vi "Init.vi"(8 "error in (no error)":errorcluster, 10 "Responder names":string[](array[string]), 11 "Response Synchronizer in":refnum<class "Response Synchronizer.lvclass">) -> (0 "error out":errorcluster, 3 "Response Synchronizer out":refnum<class "Response Synchronizer.lvclass">)   [LabVIEW 2021, in "Response Synchronizer.lvclass"]
uses:
  Response Synchronizer.lvclass
  Acquired Result/Acquired Result.lvclass
  Response Synchronizer.lvclass/Response Synchronizer.ctl
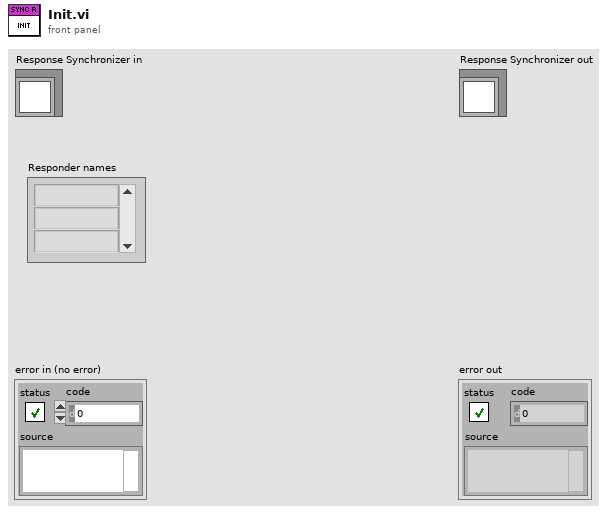
[diagram p1: front panel]
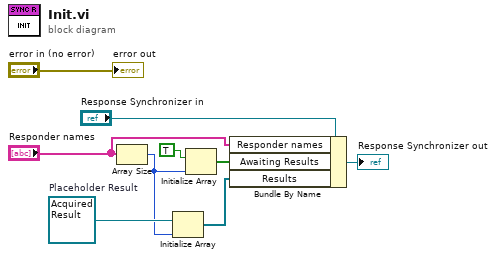
[diagram p0: block diagram]
diagram:
  w5 = refnum<class "Acquired Result.lvclass"> refnum  # Placeholder Result
  n1 = Array Size(array="Responder names") -> (size(s)=w4:i32)
  n2 = Initialize Array(w5, w4) -> (w2:refnum<class "Acquired Result.lvclass">[])
  n3 = Initialize Array(TRUE, w4) -> (w3:bool[])
  n4 = Bundle By Name(cluster="Response Synchronizer in", "Responder names"="Responder names", "Awaiting Results"=w3, "Results"=w2) -> (→"Response Synchronizer out":refnum<class "Response Synchronizer.lvclass">)
  "error out" <- "error in (no error)"
